vi "选择火焰占比系数.vi"(11 "火焰占比系数":dbl(slide)=0.9 min=0.0 max=1.0 step=0.01 scale=0.0..1.0 scale format="%1.2f") -> ()   [LabVIEW 2018]
uses:
  <vilib>/Utility/error.llb/DialogType.ctl
  <vilib>/vision/NI_Vision_Development_Module.lvlib
  Dll/fire_Otsu.dll
panel:
  in  "?":bool
  out "分割图像":T1(plugin-control)
  out "滤波平滑处理后的火焰图":T1(plugin-control)
  out "lie":i32
  out "hang":i32
  out "Histogram 3":dynamicdata(graph) caption="B直方图"
  out "Histogram 2":dynamicdata(graph) caption="A直方图"
  out "Histogram":dynamicdata(graph) caption="L直方图"
  in  "停止":bool
  out "原图":T1(plugin-control)
  # "Lab颜色空间火焰占比系数选择"
  # "火\n焰\n占\n比\n系\n数\n选\n择"
  # "火焰颜色直方图"
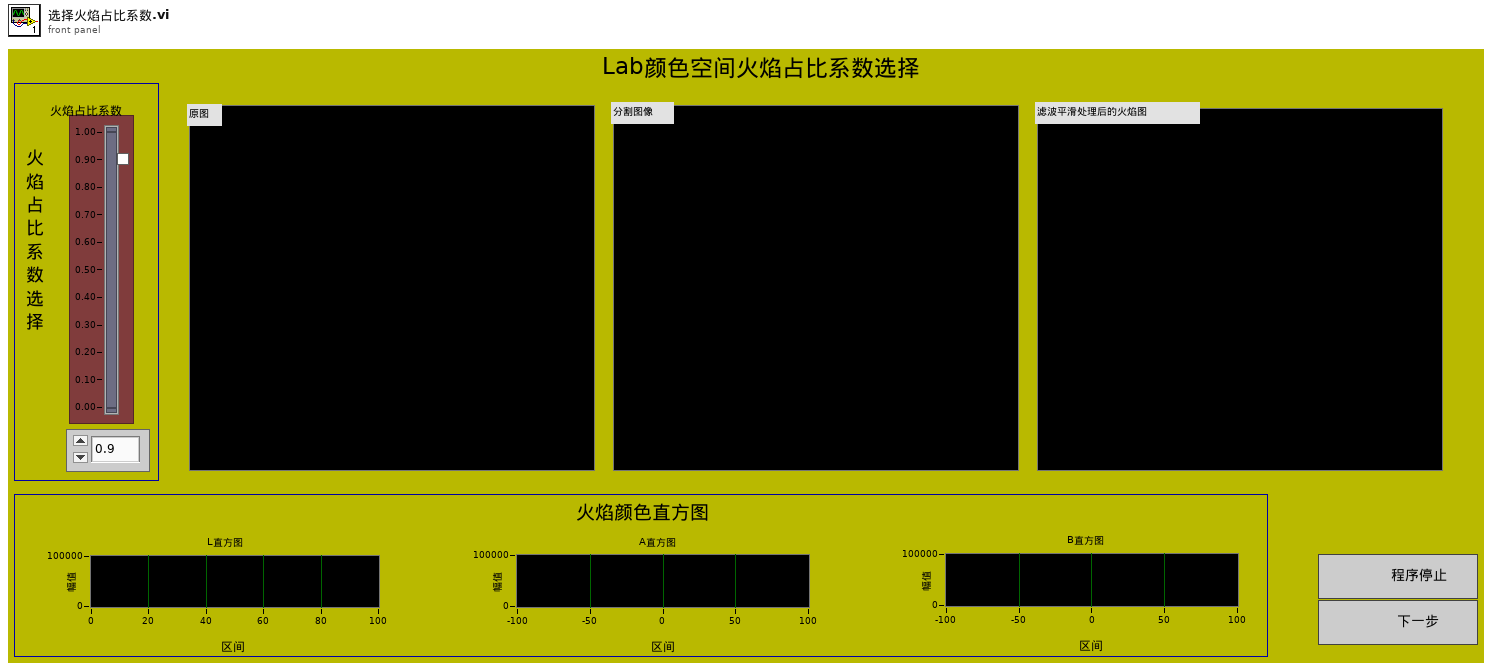
[diagram p1: front panel]
types:
  T1 = typedef "IMAQ Image.ctl" = refnum<image>
  T2 = enum8{"Enabled", "Disabled", "Disabled and Grayed Out"}
  T3 = typedef "Image Type" = u32
  T4 = typedef "DialogType.ctl" = u16
  T5 = cluster{"X Size":i32, "Y Size":i32, "% Tolerance":i32}
  T6 = typedef "ROI Descriptor" = cluster{"Global Rectangle":i32[], "Contours":cluster{"ID":enum32{"External", "Internal"}, "Type":u32, "Coordinates":i32[]}[]}
  T7 = enum32{"Invalid", "Standard", "Closed", "Hidden", "Minimized", "Maximized"}
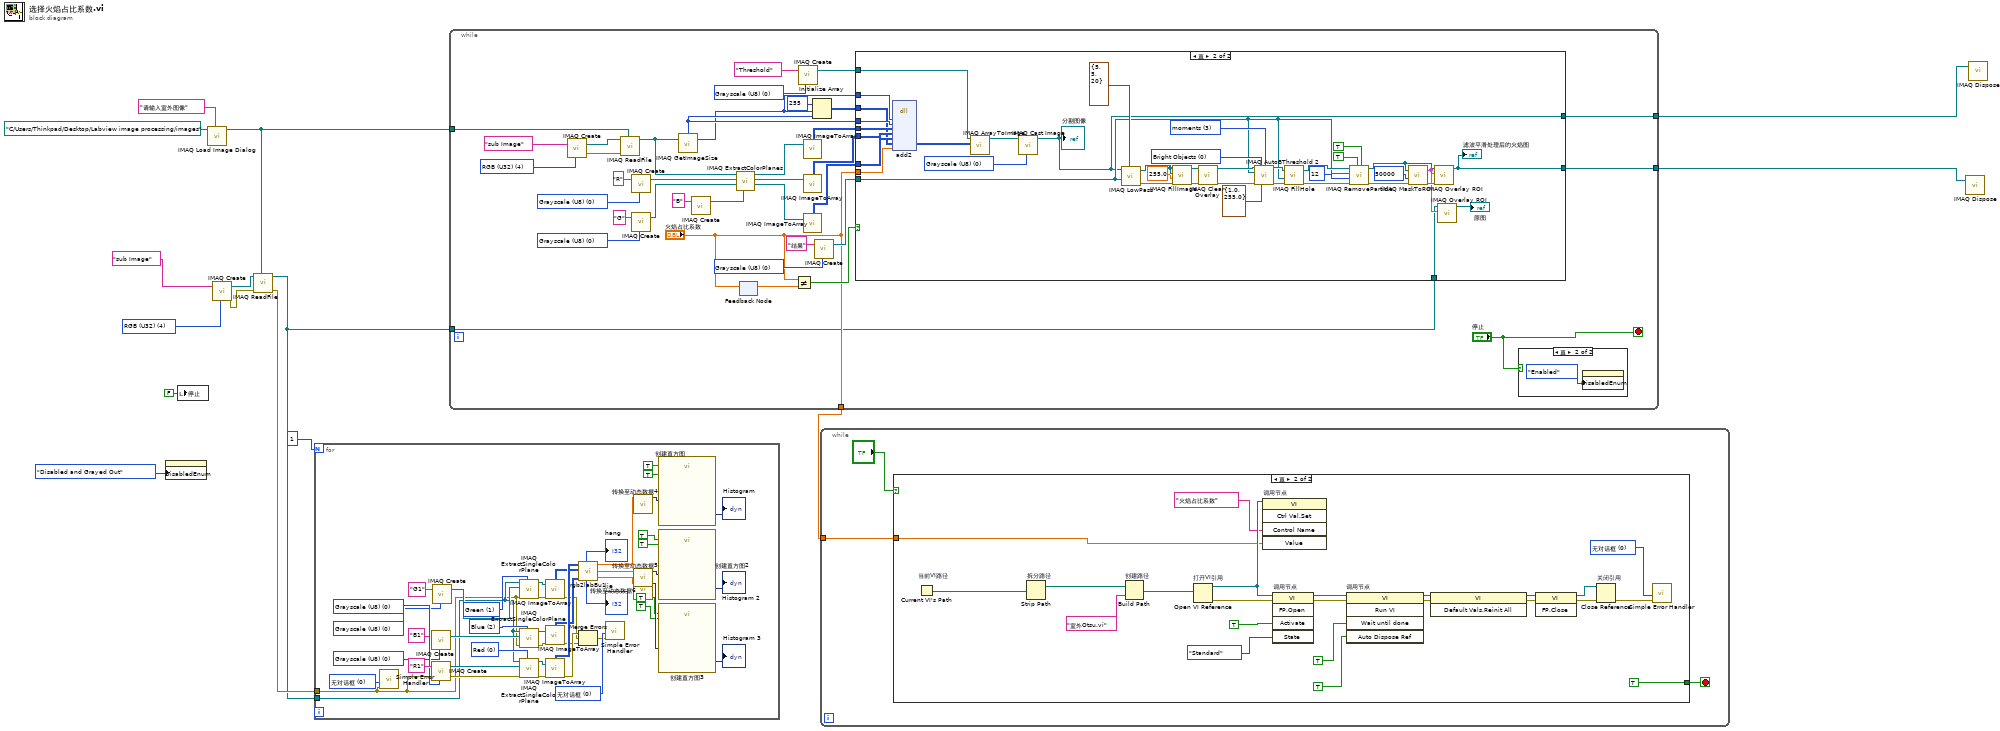
[diagram p0: block diagram]
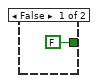
[diagram p2: hidden frame]
diagram:
  w12 = T3 4 items=["Grayscale (U8)", "Grayscale (I16)", "Grayscale (SGL)", "Complex (CSG)", "RGB (U32)", "HSL (U32)", "RGB (U64)", "Grayscale (U16)"] ("Image Type")
  n1 = property class="Bool"("DisabledEnum"=T2."Disabled and Grayed Out" ("禁用")) -> ()  [unwired: 2 in, 2 out]
  n2 = local write "停止"(FALSE ("停止")) -> ()
  n3 = call "IMAQ Load Image Dialog"("Prompt"="请输入室外图像", "Start Path"=path "C:/Users/Thinkpad/Desktop/Labview image processing/images") -> ("Path"=w10:path)  [unwired: 7 in, 2 out]
  n4 = call "IMAQ Create"("Image Name"="sub Image", "Image Type"=w12) -> ("New Image"=w11:T1, "error out"=w9:errorcluster)  [unwired: 2 in, 1 out]
  n5 = call "IMAQ ReadFile"("File Path"=w10, "error in (no error)"=w9, "Image"=w11) -> ("error out"=w6:errorcluster, "Image Out"=w3:T1)  [unwired: 4 in, 3 out]
  n6 = for {
    N: 1 -> [_]
    tunnel: w3 -> [w23]
    tunnel: w6 -> [w22]
    w27 = T4 0 items=["无对话框", "确定信息", "继续或停止信息", "确定信息＋警告", "继续/停止+警告"] ("type of dialog (OK msg:1)")
    w34 = T4 0 items=["无对话框", "确定信息", "继续或停止信息", "确定信息＋警告", "继续/停止+警告"] ("type of dialog (OK msg:1)")
    w41 = 2 items=["Red", "Green", "Blue", "Hue", "Saturation", "Luminance", "Value", "Intensity"] ("Color Plane")
    w42 = 1 items=["Red", "Green", "Blue", "Hue", "Saturation", "Luminance", "Value", "Intensity"] ("Color Plane")
    w43 = 0 items=["Red", "Green", "Blue", "Hue", "Saturation", "Luminance", "Value", "Intensity"] ("Color Plane")
    w47 = T3 0 items=["Grayscale (U8)", "Grayscale (I16)", "Grayscale (SGL)", "Complex (CSG)", "RGB (U32)", "HSL (U32)", "RGB (U64)", "Grayscale (U16)"] ("Image Type")
    w49 = T3 0 items=["Grayscale (U8)", "Grayscale (I16)", "Grayscale (SGL)", "Complex (CSG)", "RGB (U32)", "HSL (U32)", "RGB (U64)", "Grayscale (U16)"] ("Image Type")
    w51 = T3 0 items=["Grayscale (U8)", "Grayscale (I16)", "Grayscale (SGL)", "Complex (CSG)", "RGB (U32)", "HSL (U32)", "RGB (U64)", "Grayscale (U16)"] ("Image Type")
    n7 = call <vilib>:"Simple Error Handler.vi"("type of dialog (OK msg:1)"=w34, "error in (no error)"=w22) -> ()  [unwired: 3 in, 5 out]
    n8 = call "IMAQ Create"("Image Name"="B1", "Image Type"=w47) -> ("New Image"=w44:T1)  [unwired: 2 in, 2 out]
    n9 = call "IMAQ Create"("Image Name"="R1", "Image Type"=w51, "error in (no error)"=w22) -> ("New Image"=w46:T1, "error out"=w33:errorcluster)  [unwired: 1 in, 1 out]
    n10 = call "IMAQ Create"("Image Name"="G1", "Image Type"=w49) -> ("New Image"=w45:T1)  [unwired: 2 in, 2 out]
    n11 = call "IMAQ ExtractSingleColorPlane"("Color Plane"=w42, "error in (no error)"=w22, "Image Dst"=w45, "Image Src"=w23) -> ("error out"=w35:errorcluster, "Image Dst Out"=w61:T1)  [unwired: 6 in]
    n12 = call "IMAQ ExtractSingleColorPlane"("Color Plane"=w41, "error in (no error)"=w22, "Image Dst"=w44, "Image Src"=w23) -> ("error out"=w31:errorcluster, "Image Dst Out"=w60:T1)  [unwired: 6 in]
    n13 = call "IMAQ ExtractSingleColorPlane"("Color Plane"=w43, "error in (no error)"=w33, "Image Dst"=w46, "Image Src"=w23) -> ("error out"=w32:errorcluster, "Image Dst Out"=w62:T1)  [unwired: 6 in]
    n14 = call "IMAQ ImageToArray"("error in (no error)"=w35, "Image"=w61) -> ("error out"=w29:errorcluster, "Image Pixels (U8)"=w39:u8[][])  [unwired: 2 in, 3 out]
    n15 = call "IMAQ ImageToArray"("error in (no error)"=w31, "Image"=w60) -> ("error out"=w28:errorcluster, "Image Pixels (U8)"=w38:u8[][])  [unwired: 2 in, 3 out]
    n16 = call "IMAQ ImageToArray"("error in (no error)"=w32, "Image"=w62) -> ("error out"=w30:errorcluster, "Image Pixels (U8)"=w40:u8[][])  [unwired: 2 in, 3 out]
    n17 = call "rgb2labBu1.vi"("R"=w40, "G"=w39, "B"=w38) -> ("hang"=→"hang":i32, "lie"=→"lie":i32, "LZ"=w53:dbl[], "aZ"=w54:dbl[], "bZ"=w59:dbl[])  [unwired: 1 in]
    n18 = Merge Errors(w30, w29, w28) -> (w26:errorcluster)
    n19 = call <vilib>:"Simple Error Handler.vi"("type of dialog (OK msg:1)"=w27, "error in (no error)"=w26) -> ()  [unwired: 3 in, 5 out]
    n20 = call "转换至动态数据4"("Array"=w53) -> ("Dynamic Data Type"=w58:dynamicdata)  [unwired: 3 in]
    n21 = call "转换至动态数据5"("Array"=w54) -> ("Dynamic Data Type"=w57:dynamicdata)  [unwired: 3 in]
    n22 = call "转换至动态数据6"("Array"=w59) -> ("Dynamic Data Type"=w25:dynamicdata)  [unwired: 3 in]
    n23 = call "创建直方图"("Reset"=TRUE, "Enable"=TRUE, "Signal"=w58) -> ("Histogram"=→"Histogram":dynamicdata)  [unwired: 7 in, 1 out]
    n24 = call "创建直方图2"("Reset"=TRUE, "Enable"=TRUE, "Signal"=w57) -> ("Histogram"=→"Histogram 2":dynamicdata)  [unwired: 7 in, 1 out]
    n25 = call "创建直方图3"("Reset"=TRUE, "Enable"=TRUE, "Signal"=w25) -> ("Histogram"=→"Histogram 3":dynamicdata)  [unwired: 7 in, 1 out]
  }
  n26 = while {
    tunnel: w10 -> [w74]
    tunnel: [w67] -> w8
    tunnel: [w66] -> w7
    tunnel: ["火焰占比系数"] -> w4
    tunnel: w3 -> [w64]
    stop <- "停止" stop-if-true
    w69 = T3 0 items=["Grayscale (U8)", "Grayscale (I16)", "Grayscale (SGL)", "Complex (CSG)", "RGB (U32)", "HSL (U32)", "RGB (U64)", "Grayscale (U16)"] ("Image Type")
    w72 = T3 0 items=["Grayscale (U8)", "Grayscale (I16)", "Grayscale (SGL)", "Complex (CSG)", "RGB (U32)", "HSL (U32)", "RGB (U64)", "Grayscale (U16)"] ("Image Type")
    w85 = T3 0 items=["Grayscale (U8)", "Grayscale (I16)", "Grayscale (SGL)", "Complex (CSG)", "RGB (U32)", "HSL (U32)", "RGB (U64)", "Grayscale (U16)"] ("Image Type")
    w86 = T3 0 items=["Grayscale (U8)", "Grayscale (I16)", "Grayscale (SGL)", "Complex (CSG)", "RGB (U32)", "HSL (U32)", "RGB (U64)", "Grayscale (U16)"] ("Image Type")
    w97 = T3 4 items=["Grayscale (U8)", "Grayscale (I16)", "Grayscale (SGL)", "Complex (CSG)", "RGB (U32)", "HSL (U32)", "RGB (U64)", "Grayscale (U16)"] ("Image Type")
    n27 = call "IMAQ Create"("Image Name"="sub Image", "Image Type"=w97) -> ("New Image"=w98:T1, "error out"=w99:errorcluster)  [unwired: 2 in, 1 out]
    n28 = call "IMAQ ReadFile"("File Path"=w74, "error in (no error)"=w99, "Image"=w98) -> ("Image Out"=w82:T1)  [unwired: 4 in, 4 out]
    n29 = call "IMAQ Create"("Image Name"="R", "Image Type"=w86) -> ("New Image"=w93:T1)  [unwired: 3 in, 1 out]
    n30 = call "IMAQ Create"("Image Name"="G", "Image Type"=w85) -> ("New Image"=w91:T1)  [unwired: 3 in, 1 out]
    n31 = call "IMAQ GetImageSize"("Image"=w82) -> ("Y Resolution"=w80:i32, "X Resolution"=w83:i32)  [unwired: 3 in, 1 out]
    n32 = call "IMAQ Create"("Image Name"="B") -> ("New Image"=w95:T1)  [unwired: 4 in, 1 out]
    n33 = call "IMAQ ExtractColorPlanes"("Blue or Luma or Val or Inten Plane"=w95, "Green or Sat Plane"=w91, "Red or Hue Plane"=w93, "Image Src"=w82) -> ("Blue or Luma or Val or Inten Plane out"=w87:T1, "Green or Sat Plane out"=w88:T1, "Red or Hue Plane out"=w89:T1)  [unwired: 4 in, 1 out]
    n34 = feedback #1() -> (w81:dbl)  [unwired: 1 in]
    n35 = feedback-in #1("火焰占比系数") -> ()
    n36 = Not Equal?(x="火焰占比系数", y=w81) -> (x != y?=w75:bool)
    n37 = call "IMAQ Create"("Image Name"="Threshold", "Image Type"=w69) -> ("New Image"=w68:T1)  [unwired: 3 in, 1 out]
    n38 = call "IMAQ ImageToArray"("Image"=w89) -> ("Image Pixels (U8)"=w79:u8[][])  [unwired: 3 in, 4 out]
    n39 = call "IMAQ ImageToArray"("Image"=w88) -> ("Image Pixels (U8)"=w78:u8[][])  [unwired: 3 in, 4 out]
    n40 = call "IMAQ ImageToArray"("Image"=w87) -> ("Image Pixels (U8)"=w77:u8[][])  [unwired: 3 in, 4 out]
    n41 = Initialize Array ("data")(u8 255, w80, w83) -> (w76:u8[][])
    n42 = call "IMAQ Create"("Image Name"="结果", "Image Type"=w72) -> ("New Image"=w71:T1)  [unwired: 3 in, 1 out]
    n43 = case shown="真" w75 {
      tunnel: w83 -> [_ w139]
      tunnel: w80 -> [_ w116]
      tunnel: w79 -> [_ w115]
      tunnel: w78 -> [_ w114]
      tunnel: w77 -> [_ w113]
      tunnel: w76 -> [_ w112]
      tunnel: "火焰占比系数" -> [_ w111]
      tunnel: [_ w104] -> w67
      tunnel: [_ w105] -> w66
      tunnel: w68 -> [_ w109]
      tunnel: w71 -> [_ w106]
      tunnel: w64 -> [_ w102]
      frame False {
      }
      frame True {
        w107 = T3 0 items=["Grayscale (U8)", "Grayscale (I16)", "Grayscale (SGL)", "Complex (CSG)", "RGB (U32)", "HSL (U32)", "RGB (U64)", "Grayscale (U16)"] ("Image Type")
        w122 = u32 0 items=["Bright Objects", "Dark Objects"] ("Look For (Bright Objects)")
        w120 = 3 items=["clustering", "entropy", "metric", "moments", "inter-class variance"] ("Method")
        n44 = dll-call lib="PTH2Aabs DsdhProgramme_GuShiJu火焰分割Dll\nfire_Otsu.dll" fn="add2"("rows"=w116, "cols"=w139, "ImageR"=w115, "ImageG"=w114, "ImageB"=w113, "data"=w112, "a"=w111) -> ("data"=w110:u8[][])  [unwired: 10 in, 2 out]
        n45 = call "IMAQ ArrayToImage"("Image Pixels (U8)"=w110, "Image"=w109) -> ("Image Out"=w108:T1)  [unwired: 8 in, 1 out]
        n46 = call "IMAQ Cast Image"("Image Type"=w107, "Image Src"=w108) -> ("Image Dst Out"=w105:T1)  [unwired: 8 in, 1 out]
        "分割图像" <- w105
        n47 = call "IMAQ LowPass"("Image Src"=w105, "Size & Tolerance"=T5 {"X Size"=5, "Y Size"=5, "% Tolerance"=20}, "Image Dst"=w106) -> ("Image Dst Out"=w119:T1, "error out"=w134:errorcluster)  [unwired: 4 in]
        n48 = call "IMAQ FillImage"("error in (no error)"=w134, "Pixel Value (U8, U16, I16, Float)"=sgl 255.0, "Image Mask"=w119, "Image"=w119) -> ("error out"=w137:errorcluster, "Image Out"=w135:T1)  [unwired: 6 in]
        n49 = call "IMAQ Clear Overlay"("error in (no error)"=w137, "Image"=w135) -> ("error out"=w138:errorcluster, "Image Out"=w136:T1)  [unwired: 8 in]
        n50 = call "IMAQ AutoBThreshold 2"("Image Src"=w136, "Look For (Bright Objects)"=w122, "Method (clustering)"=w120, "Image Dst"=w106, "error in (no error)"=w138, "Threshold Limits"=cluster{"Lower value":sgl, "Upper value":sgl} {"Lower value"=1.0, "Upper value"=255.0}) -> ("Image Dst Out"=w133:T1, "error out"=w121:errorcluster)  [unwired: 2 in, 6 out]
        n51 = call "IMAQ FillHole"("error in (no error)"=w121, "Image Dst"=w106, "Image Src"=w133) -> ("error out"=w125:errorcluster, "Image Dst Out"=w124:T1)  [unwired: 3 in]
        n52 = call "IMAQ RemoveParticle"("Connectivity 4/8 (8)"=TRUE, "Square/Hexa (Square)"=TRUE, "error in (no error)"=w125, "Number of Erosion"=12, "Image Dst"=w106, "Image Src"=w124) -> ("error out"=w129:errorcluster, "Image Dst Out"=w130:T1)  [unwired: 4 in]
        n53 = call "IMAQ MaskToROI"("Image"=w130, "Max number of vectors in ROI"=50000, "error in (no error)"=w129) -> ("ROI Descriptor"=w103:T6, "error out"=w131:errorcluster)  [unwired: 4 in, 1 out]
        n54 = call "IMAQ Overlay ROI"("error in (no error)"=w131, "ROI Descriptor"=w103, "Image"=w130) -> ("Image Out"=w104:T1)  [unwired: 7 in, 1 out]
        "滤波平滑处理后的火焰图" <- w104
        n55 = call "IMAQ Overlay ROI"("ROI Descriptor"=w103, "Image"=w102) -> ("Image Out"=→"原图":T1)  [unwired: 8 in, 1 out]
      }
    }
    n56 = case shown="真" "停止" {
      frame False {
      }
      frame True {
        n57 = property class="Bool"("DisabledEnum"=T2."Enabled" ("禁用")) -> ()  [unwired: 2 in, 2 out]
      }
    }
  }
  n58 = while {
    tunnel: w4 -> [w141]
    stop <- w140 stop-if-true
    n59 = case shown="真" "?" {
      tunnel: w141 -> [_ w147]
      tunnel: [FALSE TRUE] -> w140
      frame False {
      }
      frame True {
        w145 = T4 0 items=["无对话框", "确定信息", "继续或停止信息", "确定信息＋警告", "继续/停止+警告"] ("type of dialog (OK msg:1)")
        n60 = Current VI's Path "当前VI路径"() -> (path=w162:path)
        n61 = Strip Path "拆分路径"(path=w162) -> (stripped path=w166:path)  [unwired: 1 out]
        n62 = Build Path "创建路径"(base path=w166, name or relative path="室外Otsu.vi" ("名称或相对路径")) -> (appended path=w163:path)
        n63 = Open VI Reference "打开VI引用"(vi path=w163) -> (vi reference=w152:refnum<vi>, error out=w160:errorcluster)  [unwired: 5 in]
        n64 = invoke on="调用节点" class="VI" method="Ctrl Val.Set"(reference=w152, "Control Name"="火焰占比系数" ("控件名"), "Value"=w147) -> ()  [unwired: 2 in, 5 out]
        n65 = invoke on="调用节点" class="VI" method="FP.Open"(reference=w152, error in=w160, "Activate"=TRUE ("激活？"), "State"=T7."Standard" ("状态")) -> (reference out=w159:refnum<vi>, error out=w158:errorcluster)  [unwired: 1 in, 3 out]
        n66 = invoke on="调用节点" class="VI" method="Run VI"(reference=w159, error in=w158, "Wait until done"=TRUE ("结束前等待"), "Auto Dispose Ref"=TRUE ("自动销毁引用")) -> (reference out=w153:refnum<vi>, error out=w155:errorcluster)  [unwired: 1 in, 3 out]
        n67 = invoke class="VI" method="Default Vals.Reinit All"(reference=w153, error in=w155) -> (reference out=w154:refnum<vi>, error out=w149:errorcluster)  [unwired: 1 in, 1 out]
        n68 = invoke class="VI" method="FP.Close"(reference=w154, error in=w149) -> (reference out=w150:refnum<vi>, error out=w148:errorcluster)  [unwired: 1 in, 1 out]
        n69 = Close Reference "关闭引用"(reference=w150, error in (no error)=w148) -> (error out=w146:errorcluster)
        n70 = call <vilib>:"Simple Error Handler.vi"("type of dialog (OK msg:1)"=w145, "error in (no error)"=w146) -> ()  [unwired: 3 in, 5 out]
      }
    }
  }
  n71 = call "IMAQ Dispose"("Image"=w8) -> ()  [unwired: 5 in, 1 out]
  n72 = call "IMAQ Dispose"("Image"=w7) -> ()  [unwired: 5 in, 1 out]
